vi "TestExec.Clear Q Tasks.vi"(10 "Exceptions":string[](array[string])=["Exit"], 11 "Q In":refnum<queue>) -> (3 "Q Out":refnum<queue>)   [LabVIEW 2019]
uses:
  <vilib>/KATE/Queues/Q.Element.ctl
  <vilib>/KATE/Queues/Queue Utils.lvlib
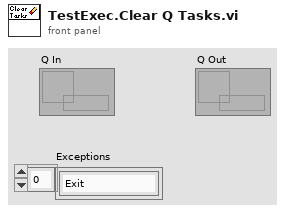
[diagram p1: front panel]
types:
  T1 = typedef "KATE_Lib.lvlib/Queue Utils.lvlib/Q.Element.ctl" = cluster{"Cmd":string, "Sub":string, "Data1":variant, "Data2":variant}
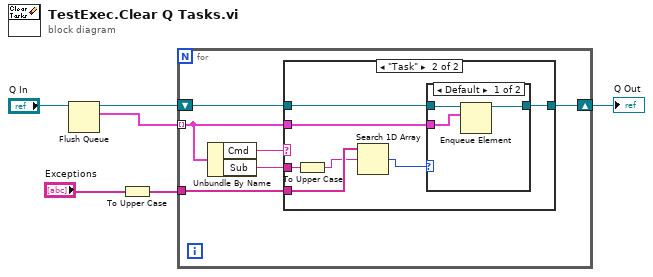
[diagram p0: block diagram]
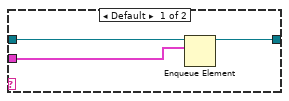
[diagram p2: hidden frame]
diagram:
  n1 = Flush Queue(queue="Q In") -> (queue out=w5:refnum<queue>, remaining elements=w6:T1[])  [unwired: 1 in, 1 out]
  n2 = To Upper Case(1:"Exceptions") -> (0:w2:string[])
  n3 = for {
    tunnel: w6 -> [w9] mode=indexing
    shift-right: [w10] -> w3
    shift-left: w5 -> [w12]
    tunnel: w2 -> [w8]
    n4 = Unbundle By Name(w9) -> ("Cmd"=w11:string, "Sub"=w7:string)
    n5 = case shown="\"Task\"" w11 {
      tunnel: w12 -> [w15 w22]
      tunnel: [w13 w18] -> w10
      tunnel: w9 -> [w14 w17]
      tunnel: w8 -> [_ w21]
      tunnel: w7 -> [_ w16]
      frame Default {
        n6 = Enqueue Element(queue=w15, element=w14) -> (queue out=w13:refnum<queue>)  [unwired: 2 in, 2 out]
      }
      frame "Task" {
        n7 = To Upper Case(1:w16) -> (0:w20:string)
        n8 = Search 1D Array(1D array=w21, element=w20) -> (index of element=w19:i32)  [unwired: 1 in]
        n9 = case shown="Default" w19 {
          tunnel: w22 -> [w25 w26]
          tunnel: [w24 w26] -> w18
          tunnel: w17 -> [w23 _]
          frame Default {
            n10 = Enqueue Element(queue=w25, element=w23) -> (queue out=w24:refnum<queue>)  [unwired: 2 in, 2 out]
          }
          frame -1 {
          }
        }
      }
    }
  }
  "Q Out" <- w3
